vi "Get Byte Count.vi"(8 "error in (no error)":errorcluster, 11 "RFFE RegWriteExt Command in":refnum<class "RFFE RegWriteExt Command.lvclass">) -> (0 "error out":errorcluster, 2 "Byte Count":i32, 3 "RFFE RegWriteExt Command out":refnum<class "RFFE RegWriteExt Command.lvclass">)   [LabVIEW 2018, in "MIPI RFFE API.lvlib" / "RFFE RegWriteExt Command.lvclass"]
uses:
  RFFE RegWriteExt Command.lvclass
  C:/Users/semoore/Projects/mipi-rffe-labview-oop/Extended Command/RFFE Extended Command.lvclass
  Extended Command/RFFE Extended Command.lvclass/RFFE Extended Command.ctl
  Extended Command/Get Register Data.vi
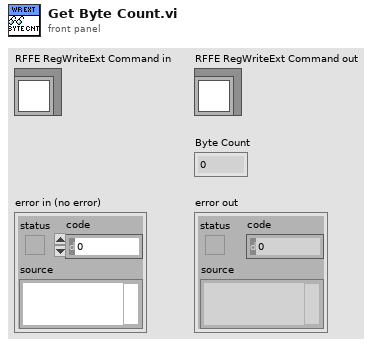
[diagram p1: front panel]
types:
  T1 = typedef "RFFE Commands.lvlib/Register Data.ctl" = u8
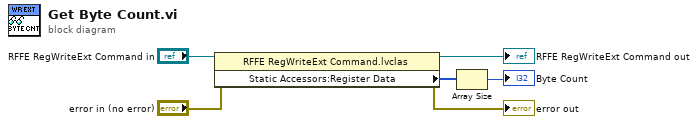
[diagram p0: block diagram]
diagram:
  n1 = property class="RFFE RegWriteExt Command.lvclas"(reference="RFFE RegWriteExt Command in", error in="error in (no error)") -> (reference out=→"RFFE RegWriteExt Command out":refnum<class "RFFE RegWriteExt Command.lvclass">, error out=→"error out":errorcluster, "Static Accessors:Register Data"=w1:T1[])
  n2 = Array Size(array=w1) -> (size(s)=→"Byte Count":i32)
